vi "Read Solenoids.vi"(8 "error in (no error)":errorcluster, 11 "Pneumatics in":refnum<class "Pneumatics.lvclass">) -> (0 "error out":errorcluster, 2 "Solenoids":T1, 3 "Pneumatics out":refnum<class "Pneumatics.lvclass">)   [LabVIEW 2019, in "Pneumatics control.lvlib" / "Pneumatics.lvclass"]
uses:
  Pneumatics.lvclass
  TypeDefs/Solenoids.ctl
  Solenoids/Solenoids.lvclass
  Pneumatics.lvclass/Pneumatics.ctl
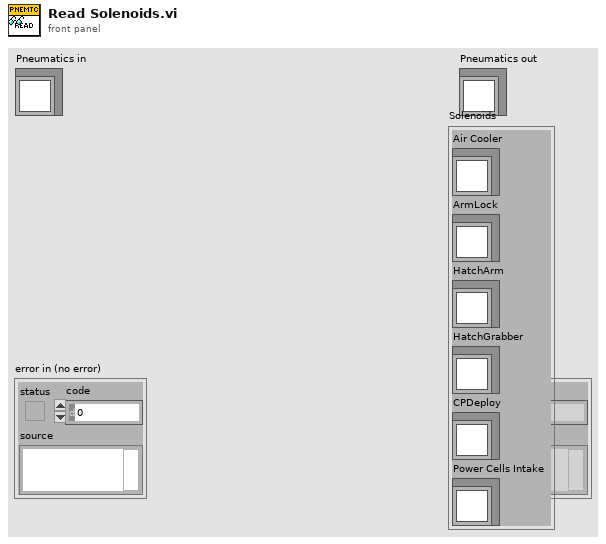
[diagram p1: front panel]
types:
  T1 = typedef "Pneumatics control.lvlib/Pneumatics.lvclass/Solenoids.ctl" = cluster{"Air Cooler":refnum<class "Solenoids.lvclass">, "ArmLock":refnum<class "Solenoids.lvclass">, "HatchArm":refnum<class "Solenoids.lvclass">, "HatchGrabber":refnum<class "Solenoids.lvclass">, "CPDeploy":refnum<class "Solenoids.lvclass">, "Power Cells Intake":refnum<class "Solenoids.lvclass">}
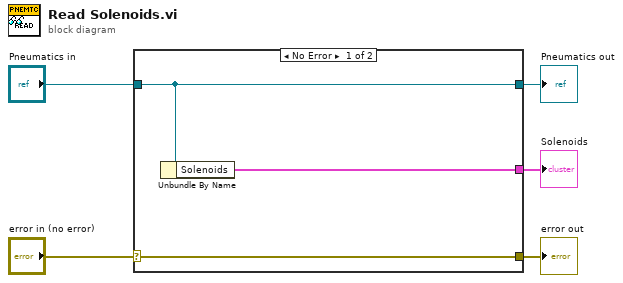
[diagram p0: block diagram]
diagram:
  n1 = case shown="No Error" "error in (no error)" {
    selector: "error in (no error)" -> [w8 w9]
    tunnel: [w8 w9] -> w4
    tunnel: [w7 w10] -> w2
    tunnel: "Pneumatics in" -> [w7 w10]
    tunnel: [w6 _] -> w1
    frame No Error {
      n2 = Unbundle By Name(w7) -> ("Solenoids"=w6:T1)
    }
    frame Error {
    }
  }
  "error out" <- w4
  "Pneumatics out" <- w2
  "Solenoids" <- w1
